vi "PercentDifference.vi"(2 "CompareeArray":dbl[](array[numeric]), 3 "Basis":dbl, 4 "Comparee":dbl) -> (0 "PercentageDifferenceArray":dbl[](array[numeric]), 1 "PercentageDifference":dbl)   [LabVIEW 2012]
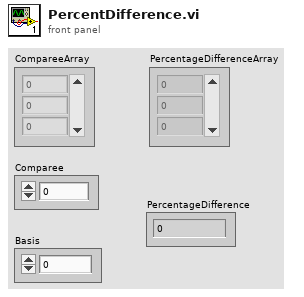
[diagram p1: front panel]
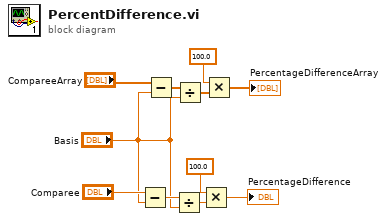
[diagram p0: block diagram]
diagram:
  n1 = Subtract(x="Comparee", y="Basis") -> (x-y=w7:dbl)
  n2 = Subtract(x="CompareeArray", y="Basis") -> (x-y=w6:dbl[])
  n3 = Divide(x=w7, y="Basis") -> (x/y=w8:dbl)
  n4 = Divide(x=w6, y="Basis") -> (x/y=w5:dbl[])
  n5 = Multiply(x=100.0 ("y"), y=w8) -> (x*y=→"PercentageDifference":dbl)
  n6 = Multiply(x=100.0 ("y"), y=w5) -> (x*y=→"PercentageDifferenceArray":dbl[])
